vi "Hypervisor.vi"() -> ()   [LabVIEW 2014]
uses:
  HypervisorState.ctl
  Resource.ctl
  Resource Type.ctl
  Sensor Reading.ctl
  <vilib>/NI/Tools/String/Tools_String.lvlib
panel:
  out "Terminal":string
  in  "Module DataType 2":T1
  in  "Cancel Button":bool
  in  "Load Settings":bool
  in  "Config File":path=path "C:/developer/New Model/config.txt"
  in  "Hypervisor State":T3=enum."Hypervisor.Sleeping"
  # "This is the hypervisor VI - it reads in a config file and loads the sub-VI's dictated in it asynchronously."
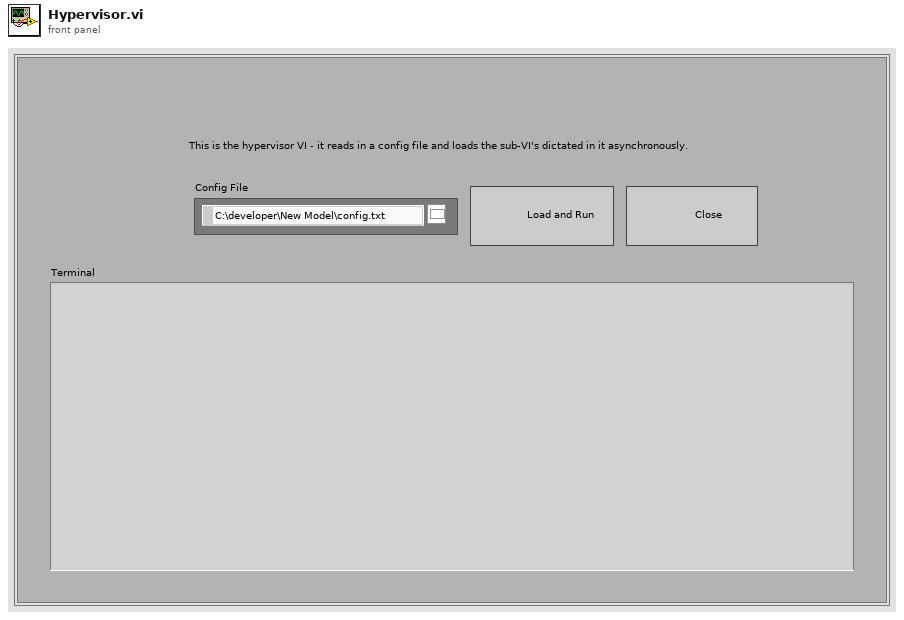
[diagram p1: front panel]
types:
  T1 = typedef "Resource.ctl" = cluster{"Module Name":string, "Message Queue":refnum<queue>, "Resource Type":T2, "Current State":enum16{"Invalid", "InMemory", "Running", "Paused", "Error", ""}, "Data Queue":refnum<queue>, "VI Reference":refnum<vi>}
  T2 = typedef "Resource Type.ctl" = enum16{"Consumer", "Producer", "Observer"}
  T3 = typedef "HypervisorState.ctl" = enum16{"Hypervisor.Error", "Hypervisor.Sleeping", "Hypervisor.Loaded", "Hypervisor.Booting", "Hypervisor.Testing", "Hypervisor.Calibrating", "Hypervisor.Running"}
  T4 = enum16{"Invalid", "InMemory", "Running", "Paused", "Error", ""}
  T5 = typedef "Config Data.ctl" = cluster{"Tower ID":string, "Access Password":string, "Modules to Load":path[]}
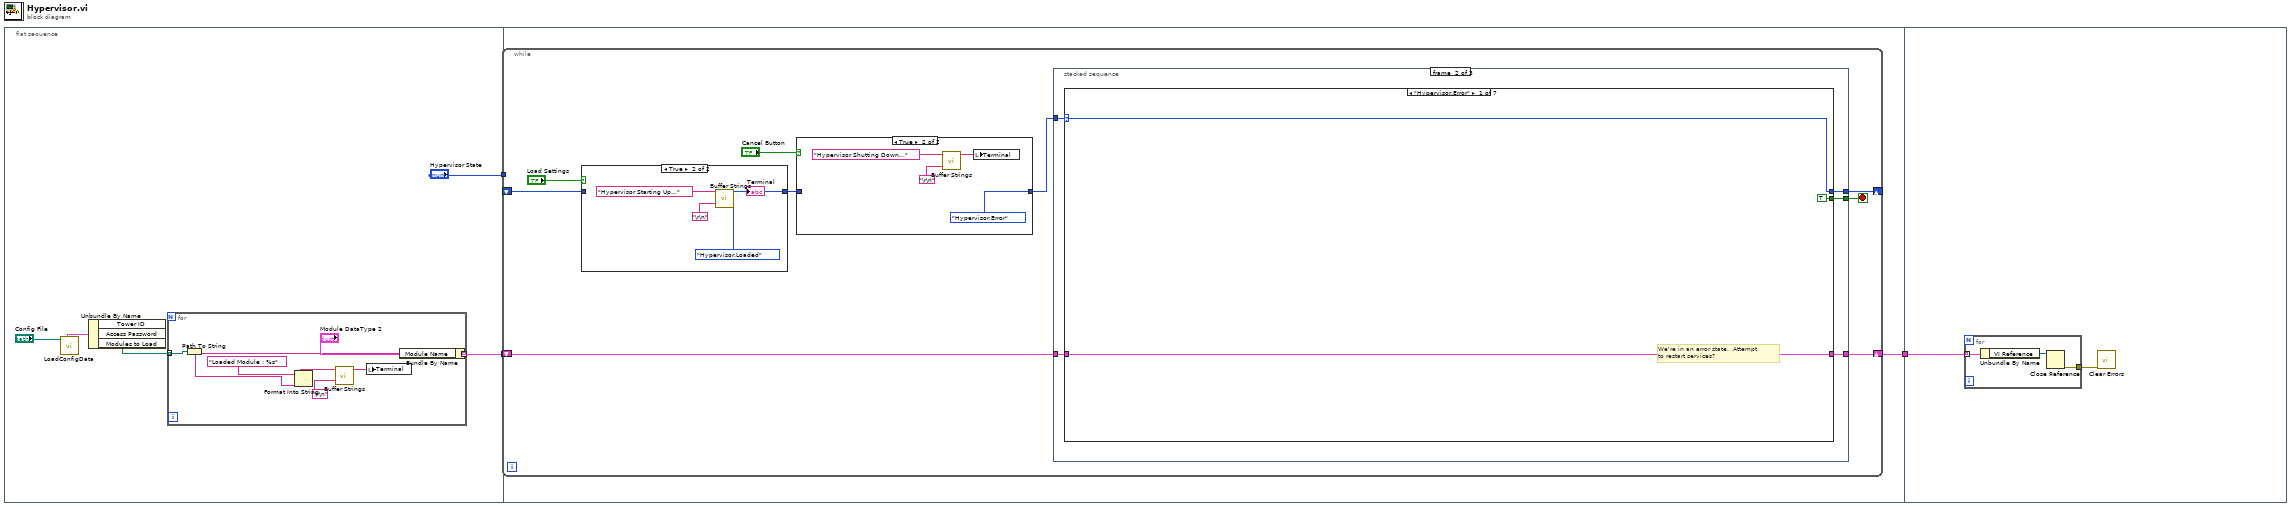
[diagram p0: block diagram]
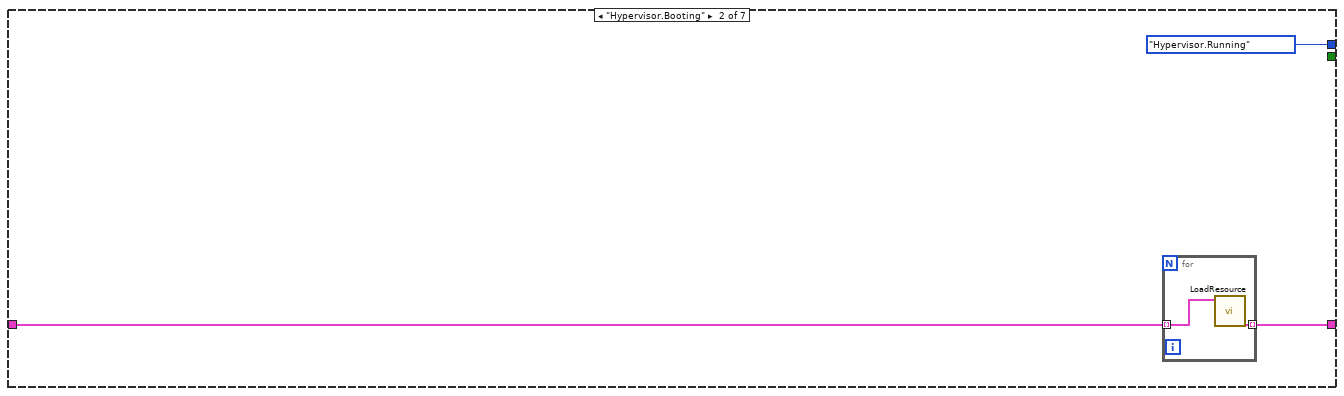
[diagram p5: hidden frame]
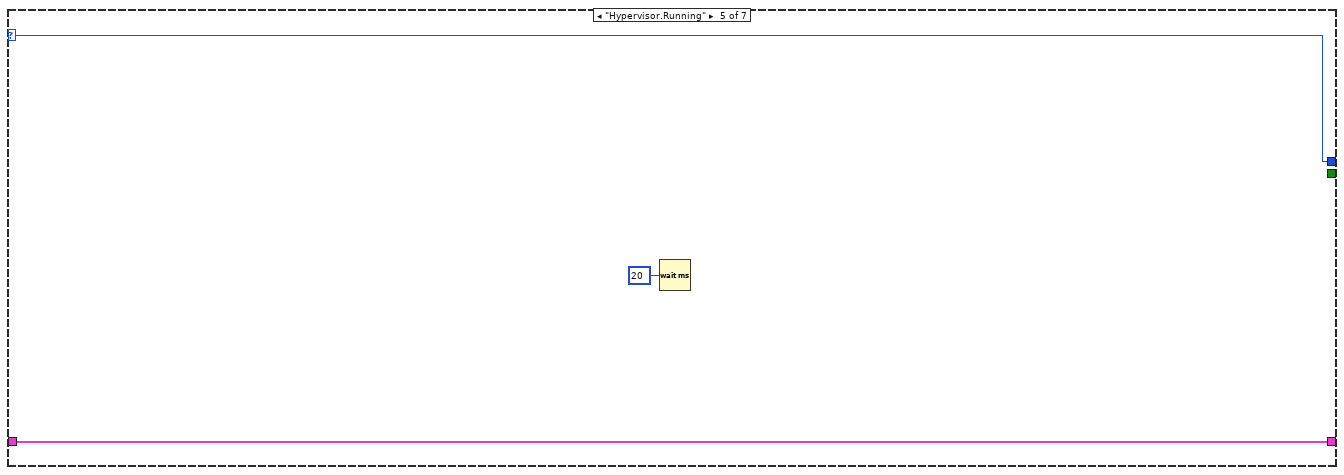
[diagram p8: hidden frame]
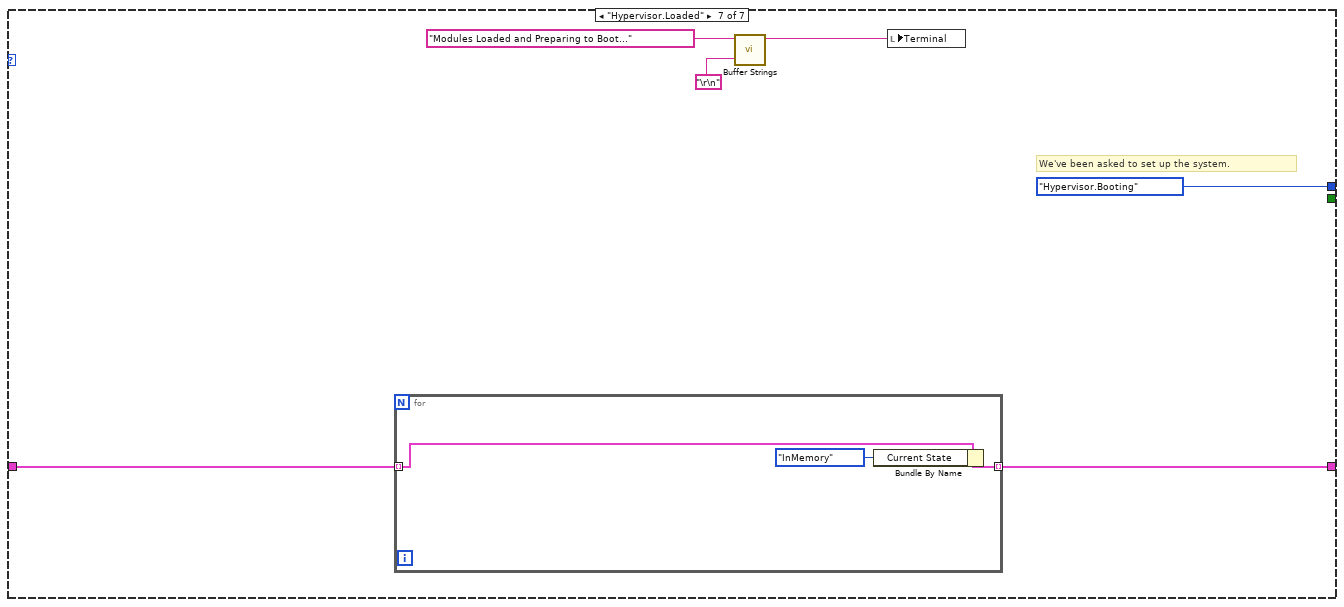
[diagram p10: hidden frame]
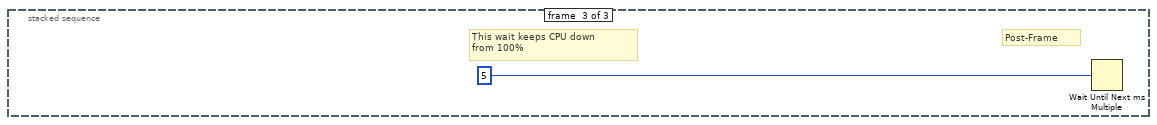
[diagram p11: hidden frame]
diagram:
  n1 = flat-sequence {
    tunnel: ["Hypervisor State"] -> w3
    tunnel: [w5] -> w2
    tunnel: w3 -> [w19]
    tunnel: w2 -> [w18]
    tunnel: [w17] -> w1
    tunnel: w1 -> [w72]
    frame #0 {
      n2 = call "LoadConfigData.vi"("Config File in"="Config File") -> ("Config Data out"=w6:T5)  [unwired: 10 in]
      n3 = Unbundle By Name(w6) -> ("Modules to Load"=w4:path[])  [unwired: 2 out]
      n4 = for {
        tunnel: w4 -> [w10] mode=indexing
        tunnel: [w15] -> w5 mode=indexing
        n5 = Path To String(path=w10) -> (string=w9:string)
        n6 = Format Into String(format string="Loaded Module : %s", w9) -> (resulting string=w14:string)  [unwired: 2 in, 1 out]
        n7 = call <vilib>:"Buffer Strings.vi"("Insert between Strings (\"\")"="\r\n", "new string"=w14) -> ("buffered string series"=w12:string)  [unwired: 9 in]
        n8 = local write "Terminal"(w12) -> ()
        n9 = Bundle By Name(cluster="Module DataType 2", "Module Name"=w9) -> (w15:T1)
      }
    }
    frame #1 {
      n10 = while {
        shift-right: [w27] -> w17
        shift-left: w18 -> [w28]
        shift-right: [w26] -> _
        shift-left: w19 -> [w24]
        stop <- w25 stop-if-true
        n11 = case shown="True" "Load Settings" {
          tunnel: w24 -> [w34 _]
          tunnel: [w34 HypervisorState."Hypervisor.Loaded" ("Hypervisor State")] -> w22
          frame False {
          }
          frame True {
            n12 = call <vilib>:"Buffer Strings.vi"("Insert between Strings (\"\")"="\r\n", "new string"="Hypervisor Starting Up...") -> ("buffered string series"=→"Terminal":string)  [unwired: 9 in]
          }
        }
        n13 = case shown="True" "Cancel Button" {
          tunnel: w22 -> [w29 _]
          tunnel: [w29 HypervisorState."Hypervisor.Error" ("Hypervisor State")] -> w21
          frame False {
          }
          frame True {
            n14 = call <vilib>:"Buffer Strings.vi"("Insert between Strings (\"\")"="\r\n", "new string"="Hypervisor Shutting Down...") -> ("buffered string series"=w30:string)  [unwired: 9 in]
            n15 = local write "Terminal"(w30) -> ()
          }
        }
        n16 = stacked-sequence {
          tunnel: w21 -> [_ w40 _]
          tunnel: w28 -> [_ w43 _]
          tunnel: [_ w42 _] -> w27
          tunnel: [_ w41 _] -> w26
          tunnel: [_ w39 _] -> w25
          frame #0 {
            # "Pre-Frame"
          }
          frame #1 {
            n17 = case shown="\"Hypervisor.Error\"" w40 {
              selector: w40 -> [w45 _ w52 w54 w58 w59 _]
              tunnel: w43 -> [w46 w49 w53 w55 w57 w60 w66]
              tunnel: [w46 w48 w53 w55 w57 w60 w65] -> w42
              tunnel: [w45 HypervisorState."Hypervisor.Running" ("Hypervisor State") w52 w54 w58 w59 HypervisorState."Hypervisor.Booting" ("Hypervisor State")] -> w41
              tunnel: [TRUE _ _ _ _ _ _] -> w39
              frame "Hypervisor.Error" {
                # "We're in an error state.  Attempt\nto restart services?"
              }
              frame "Hypervisor.Booting" {
                n18 = for {
                  tunnel: w49 -> [w51] mode=indexing
                  tunnel: [w50] -> w48 mode=indexing
                  n19 = call "LoadResource.vi"("Resource in"=w51) -> ("Resource out"=w50:T1)  [unwired: 9 in, 1 out]
                }
              }
              frame "Hypervisor.Testing" {
              }
              frame "Hypervisor.Calibrating" {
              }
              frame "Hypervisor.Running" {
                n20 = Wait (ms)(milliseconds to wait=u32 20) -> ()  [unwired: 1 out]
              }
              frame "Hypervisor.Sleeping" {
                # "Do Nothing."
              }
              frame "Hypervisor.Loaded" {
                # "We've been asked to set up the system."
                n21 = for {
                  tunnel: [w69] -> w65 mode=indexing
                  tunnel: w66 -> [w68] mode=indexing
                  n22 = Bundle By Name(cluster=w68, "Current State"=T4."InMemory") -> (w69:T1)
                }
                n23 = call <vilib>:"Buffer Strings.vi"("Insert between Strings (\"\")"="\r\n", "new string"="Modules Loaded and Preparing to Boot...") -> ("buffered string series"=w61:string)  [unwired: 9 in]
                n24 = local write "Terminal"(w61) -> ()
              }
            }
          }
          frame #2 {
            # "This wait keeps CPU down\nfrom 100%"
            # "Post-Frame"
            n25 = Wait Until Next ms Multiple(millisecond multiple=u32 5) -> ()  [unwired: 1 out]
          }
        }
      }
    }
    frame #2 {
      n26 = for {
        tunnel: w72 -> [w75] mode=indexing
        tunnel: [w73] -> w71
        n27 = Unbundle By Name(w75) -> ("VI Reference"=w74:refnum<vi>)
        n28 = Close Reference(reference=w74) -> (error out=w73:errorcluster)  [unwired: 1 in]
      }
      n29 = call <vilib>:"Clear Errors.vi"("error in (no error)"=w71) -> ()  [unwired: 5 in, 2 out]
    }
  }
